vi "Serial Data To String.vi"(4 "Serial Data":T1) -> (1 "serial data string":string)   [LabVIEW 2025]
uses:
  Serial Data.ctl
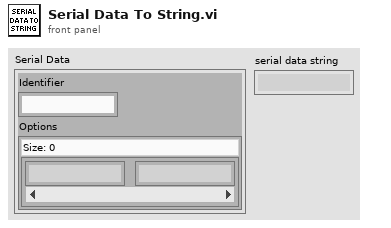
[diagram p1: front panel]
types:
  T1 = typedef "Serial Data.ctl" = cluster{"Identifier":string, "Options":map{string, string}}
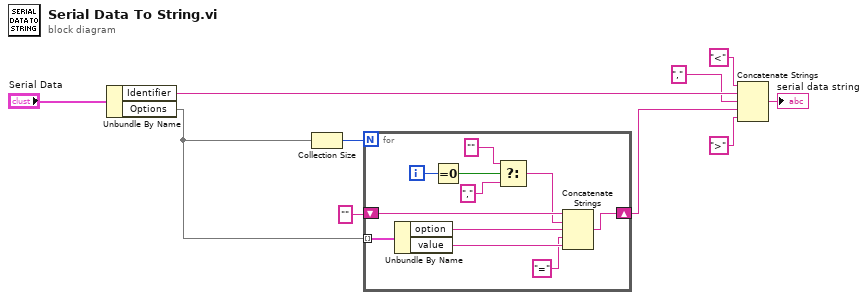
[diagram p0: block diagram]
diagram:
  n1 = Unbundle By Name("Serial Data") -> ("Identifier"=w5:string, "Options"=w4:map{string, string})
  n2 = Collection Size(1:w4) -> (0:w10:i32)
  n3 = for {
    N: w10 -> [_]
    shift-right: [w11] -> w3
    shift-left: "" -> [w17]
    tunnel: w4 -> [w21] mode=indexing
    i -> [w16]
    n4 = Unbundle By Name(w21) -> ("option"=w20:string, "value"=w19:string)
    n5 = Equal To 0?(x=w16) -> (x = 0?=w15:bool)
    n6 = Select(t="", s=w15, f=",") -> (s? t:f=w12:string)
    n7 = Concatenate Strings(w17, w12, w20, "=" ("string"), w19) -> (w11:string)
  }
  n8 = Concatenate Strings("<" ("string"), w5, "," ("string"), w3, ">" ("string")) -> (→"serial data string":string)
